vi "PickNumber.vi"(10 "Second Number":dbl, 11 "First Number":dbl) -> (2 "Y Out":dbl, 3 "X Out":dbl)   [LabVIEW 2014]
panel:
  in  "OK Button":bool
  # "Enter Two Numbers"
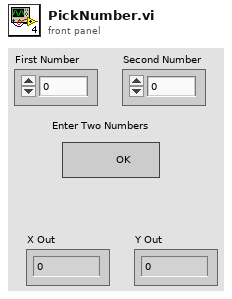
[diagram p1: front panel]
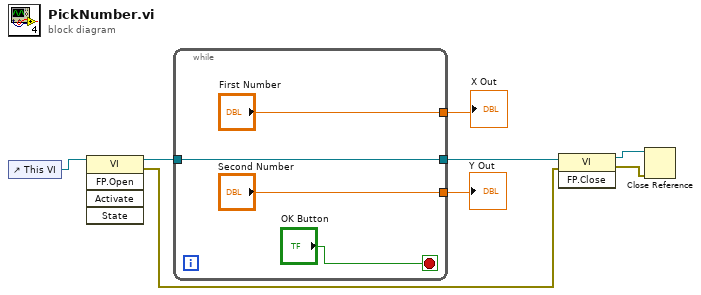
[diagram p0: block diagram]
diagram:
  n1 = control-ref of="This VI"() -> (w6:refnum<vi>)
  n2 = invoke class="VI" method="FP.Open"(reference=w6) -> (reference out=w5:refnum<vi>, error out=w1:errorcluster)  [unwired: 4 in, 3 out]
  n3 = while {
    tunnel: ["First Number"] -> w8
    tunnel: ["Second Number"] -> w7
    tunnel: w5 -> [w9]
    tunnel: [w9] -> w4
    stop <- "OK Button" stop-if-true
  }
  "X Out" <- w8
  "Y Out" <- w7
  n4 = invoke class="VI" method="FP.Close"(reference=w4, error in=w1) -> (reference out=w3:refnum<vi>, error out=w2:errorcluster)  [unwired: 1 in, 1 out]
  n5 = Close Reference(reference=w3, error in (no error)=w2) -> ()  [unwired: 1 out]
